vi "Init Pressure Transducers.vi"() -> (0 "Error Out":errorcluster, 3 "task out":refnum<k21>)   [LabVIEW 2018]
uses:
  <vilib>/DAQmx/create/channels.llb/DAQmx Create Channel (AI-Current-Basic).vi
  <vilib>/DAQmx/configure/timing.llb/DAQmx Timing (Sample Clock).vi
  <resource>/objmgr/daqmx.rc
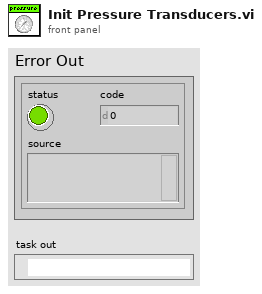
[diagram p1: front panel]
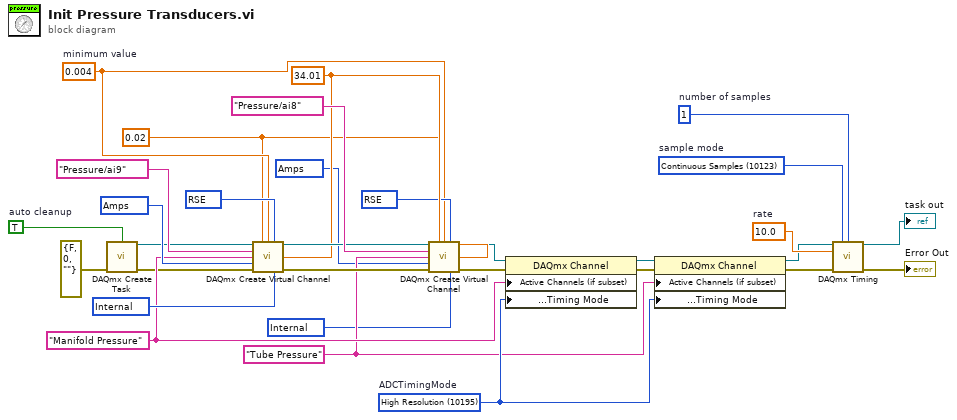
[diagram p0: block diagram]
diagram:
  w3 = TRUE  # auto cleanup
  w10 = 10123 items=["Finite Samples"=10178, "Continuous Samples"=10123, "Hardware Timed Single Point"=12522]  # sample mode
  w9 = 1  # number of samples
  w11 = 10.0  # rate
  w14 = 10200 items=["default"=-1, "Internal"=10200, "External"=10167] ("shunt resistor location")
  w15 = 10342 items=["Amps"=10342, "From Custom Scale"=10065] ("units")
  w16 = 10083 items=["default"=-1, "RSE"=10083, "NRSE"=10078, "Differential"=10106, "Pseudodifferential"=12529] ("input terminal configuration")
  w20 = 10195 items=["High Resolution"=10195, "High Speed"=14712, "Best 50 Hz Rejection"=14713, "Best 60 Hz Rejection"=14714]  # ADCTimingMode
  w19 = "Tube Pressure" ("name to assign")
  w21 = "Manifold Pressure" ("name to assign")
  w25 = 34.01 ("external shunt resistor value")
  w24 = 10200 items=["default"=-1, "Internal"=10200, "External"=10167] ("shunt resistor location")
  w30 = 10083 items=["default"=-1, "RSE"=10083, "NRSE"=10078, "Differential"=10106, "Pseudodifferential"=12529] ("input terminal configuration")
  w13 = 0.004  # minimum value
  w12 = 0.02 ("maximum value")
  w28 = 10342 items=["Amps"=10342, "From Custom Scale"=10065] ("units")
  n1 = call <vilib>:"DAQmx Create Task.vi"("auto cleanup"=w3, "error in"=errorcluster {"status"=FALSE, "code"=0, "source"=""}) -> ("task out"=w1:refnum<k21>, "error out"=w2:errorcluster)  [unwired: 12 in]
  n2 = call-poly <vilib>:"DAQmx Create Virtual Channel.vi"("task in"=w1, "maximum value"=w12, "minimum value"=w13, "input terminal configuration"=w30, "physical channels"=tag "Pressure/ai9", "name to assign"=w21, "external shunt resistor value"=w25, "units"=w28, "error in"=w2, "shunt resistor location"=w24) -> ("task out"=w26:refnum<k21>, "error out"=w27:errorcluster)  [unwired: 4 in]
  n3 = call-poly <vilib>:"DAQmx Create Virtual Channel.vi"("task in"=w26, "maximum value"=w12, "minimum value"=w13, "input terminal configuration"=w16, "physical channels"=tag "Pressure/ai8", "name to assign"=w19, "external shunt resistor value"=w25, "units"=w15, "error in"=w27, "shunt resistor location"=w14) -> ("task out"=w18:refnum<k21>, "error out"=w17:errorcluster)  [unwired: 4 in]
  n4 = property class="DAQmx Channel"(reference=w18, error in=w17, "Active Channels (if subset)"=w21, "Analog Input:General Properties:Digitizer/ADC:Timing Mode"=w20) -> (reference out=w22:refnum<k21>, error out=w23:errorcluster)
  n5 = property class="DAQmx Channel"(reference=w22, error in=w23, "Active Channels (if subset)"=w19, "Analog Input:General Properties:Digitizer/ADC:Timing Mode"=w20) -> (reference out=w6:refnum<k21>, error out=w8:errorcluster)
  n6 = call-poly <vilib>:"DAQmx Timing.vi"("task/channels in"=w6, "sample mode"=w10, "samples per channel"=w9, "rate"=w11, "error in"=w8) -> ("task out"=→"task out":refnum<k21>, "error out"=→"Error Out":errorcluster)  [unwired: 9 in]
